vi "Configure Measurement Range.vi"(0 "VISA resource name":refnum<visa-resource-name>, 1 "Current Range (0.1 A)":dbl=0.1, 2 "Minimum Current Range (0.1 A)":dbl=0.1, 5 "Source Measure Unit Channel (0: Channel A)":i32(ring) items=["Channel A", "Channel B"], 7 "Range Type (0: Current)":i32(ring) items=["Current", "Voltage"], 9 "Range Mode (1: Auto Range On)":i32(ring)=1 items=["Auto Range Off", "Auto Range On", "Auto Range Follow Limit"], 11 "error in (no error)":errorcluster, 12 "Voltage Range (0.2 V)":dbl=0.2, 13 "Minimum Voltage Range (0.2 V)":dbl=0.2) -> (4 "VISA resource name out":refnum<visa-resource-name>, 15 "error out":errorcluster)   [LabVIEW 2019, in "Keithley 2600 Series.lvlib"]
doc: "Configures the measurement range for voltage or current."
uses:
  Keithley 2600 Series.lvlib
panel:
  # "Auto Range Off"
  # "Auto Range On"
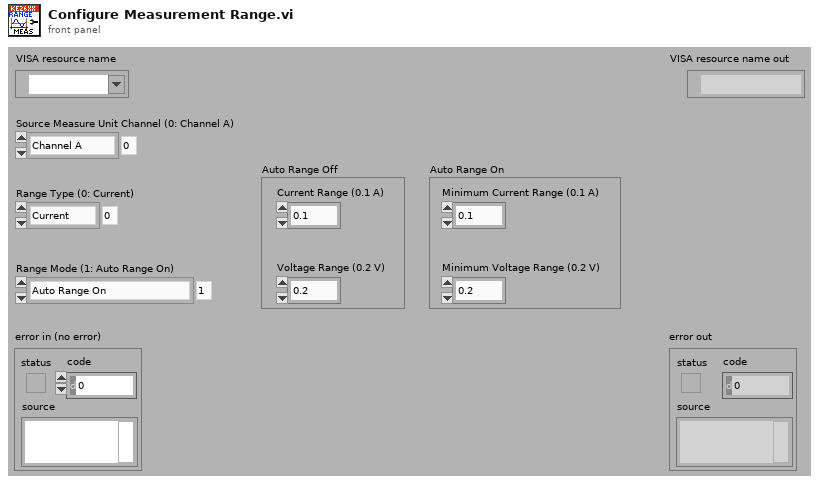
[diagram p1: front panel]
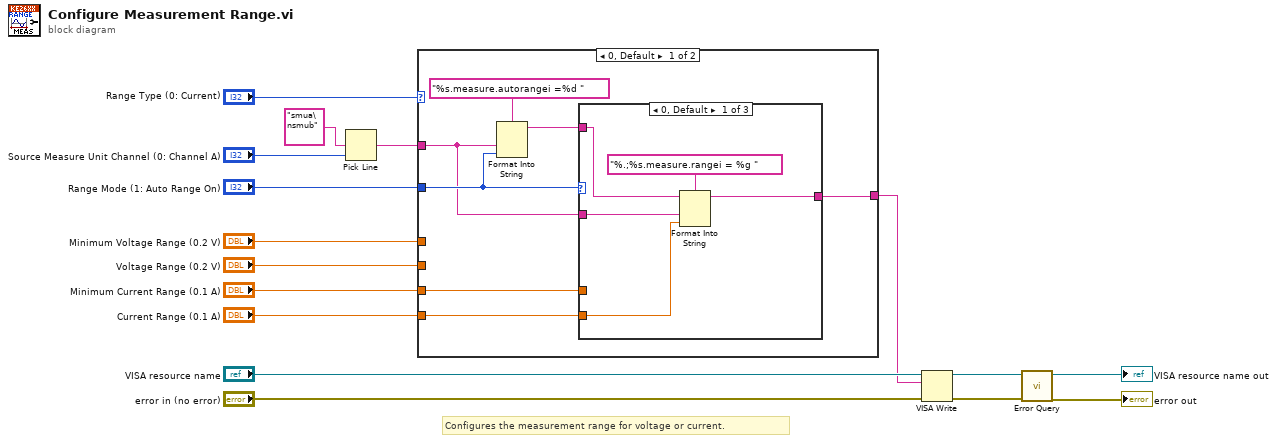
[diagram p0: block diagram]
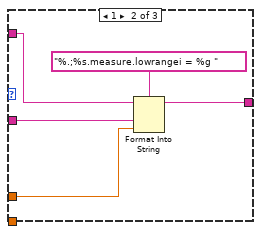
[diagram p2: hidden frame]
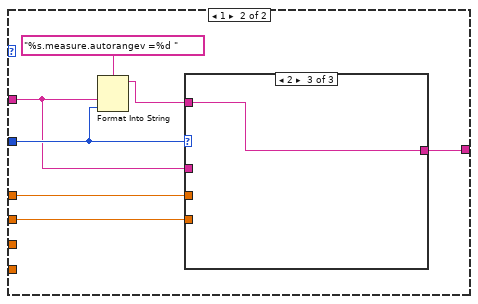
[diagram p4: hidden frame]
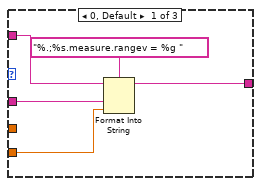
[diagram p5: hidden frame]
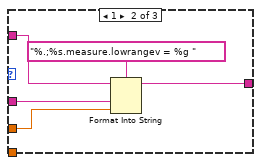
[diagram p6: hidden frame]
diagram:
  # "Configures the measurement range for voltage or current."
  n1 = Pick Line(multi-line string="smua\nsmub", line index="Source Measure Unit Channel (0: Channel A)") -> (output string=w6:string)  [unwired: 1 in]
  n2 = case shown="0, Default" "Range Type (0: Current)" {
    tunnel: "Range Mode (1: Auto Range On)" -> [w21 w40]
    tunnel: w6 -> [w20 w39]
    tunnel: "Minimum Voltage Range (0.2 V)" -> [_ w38]
    tunnel: "Voltage Range (0.2 V)" -> [_ w37]
    tunnel: "Minimum Current Range (0.1 A)" -> [w19 _]
    tunnel: "Current Range (0.1 A)" -> [w18 _]
    tunnel: [w17 w36] -> w1
    frame 0, Default {
      n3 = Format Into String(format string="%s.measure.autorangei =%d ", w20, w21) -> (resulting string=w22:string)  [unwired: 2 in, 1 out]
      n4 = case shown="0, Default" w21 {
        tunnel: w22 -> [w24 w29 w34]
        tunnel: w20 -> [w27 w33 _]
        tunnel: w19 -> [_ w32 _]
        tunnel: w18 -> [w26 _ _]
        tunnel: [w25 w30 w34] -> w17
        frame 0, Default {
          n5 = Format Into String(format string="%.;%s.measure.rangei = %g ", initial string=w24, w27, w26) -> (resulting string=w25:string)  [unwired: 1 in, 1 out]
        }
        frame 1 {
          n6 = Format Into String(format string="%.;%s.measure.lowrangei = %g ", initial string=w29, w33, w32) -> (resulting string=w30:string)  [unwired: 1 in, 1 out]
        }
        frame 2 {
        }
      }
    }
    frame 1 {
      n7 = Format Into String(format string="%s.measure.autorangev =%d ", w39, w40) -> (resulting string=w35:string)  [unwired: 2 in, 1 out]
      n8 = case shown="2" w40 {
        tunnel: w39 -> [w45 w48 _]
        tunnel: w38 -> [_ w49 _]
        tunnel: w37 -> [w44 _ _]
        tunnel: [w43 w47 w52] -> w36
        tunnel: w35 -> [w42 w50 w52]
        frame 0, Default {
          n9 = Format Into String(format string="%.;%s.measure.rangev = %g ", initial string=w42, w45, w44) -> (resulting string=w43:string)  [unwired: 1 in, 1 out]
        }
        frame 1 {
          n10 = Format Into String(format string="%.;%s.measure.lowrangev = %g ", initial string=w50, w48, w49) -> (resulting string=w47:string)  [unwired: 1 in, 1 out]
        }
        frame 2 {
        }
      }
    }
  }
  n11 = VISA Write(VISA resource name="VISA resource name", write buffer=w1, error in (no error)="error in (no error)") -> (VISA resource name out=w14:refnum<visa-resource-name>, error out=w13:errorcluster)  [unwired: 1 out]
  n12 = call "Error Query.vi"("error in (no error)"=w13, "VISA resource name"=w14) -> ("error out"=→"error out":errorcluster, "VISA resource name out"=→"VISA resource name out":refnum<visa-resource-name>)  [unwired: 6 in, 2 out]
